vi "复制模板.vi"(8 "error in":errorcluster, 10 "服务器地址":path, 11 "工单号":string) -> (0 "error out":errorcluster, 1 "参数存储地址":path, 3 "source path out":path)   [LabVIEW 2016]
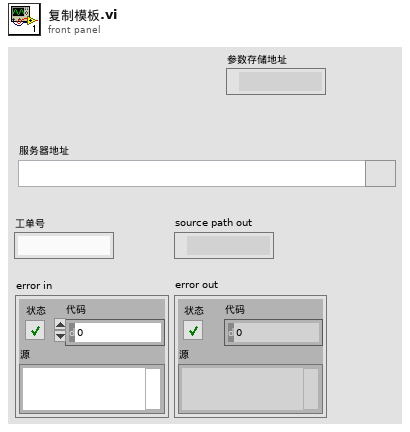
[diagram p1: front panel]
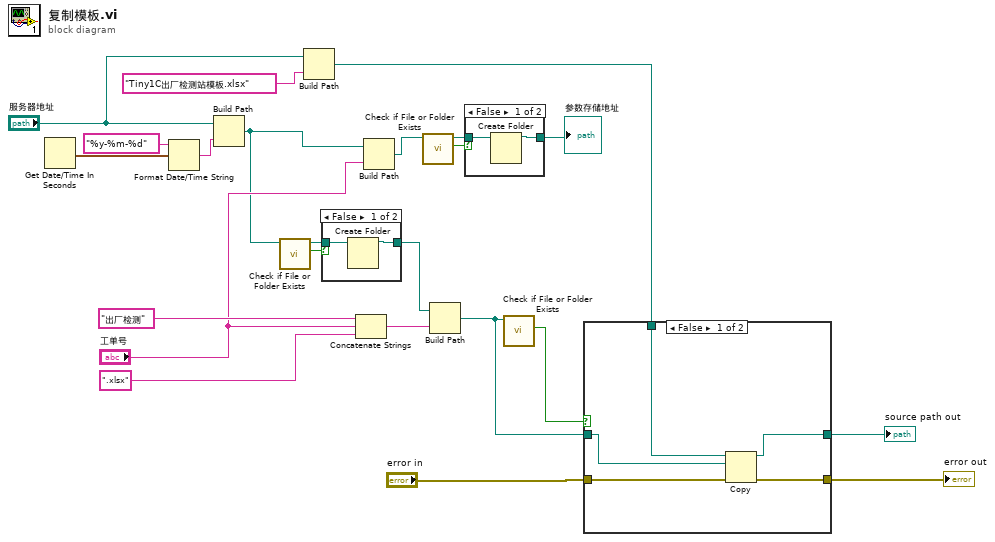
[diagram p0: block diagram]
diagram:
  n1 = Get Date/Time In Seconds() -> (seconds since 1Jan1904=w13:timestamp)
  n2 = Format Date/Time String(time format string (%c)="%y-%m-%d", seconds (now)=w13) -> (date/time string=w11:string)  [unwired: 1 in]
  n3 = Build Path(base path="服务器地址", name or relative path=w11) -> (appended path=w6:path)
  n4 = call <vilib>:"Check if File or Folder Exists.vi"("path"=w6) -> ("file or folder exists?"=w8:bool, "dup path"=w9:path)  [unwired: 8 in, 1 out]
  n5 = Build Path(base path="服务器地址", name or relative path="Tiny1C出厂检测站模板.xlsx") -> (appended path=w14:path)
  n6 = case shown="False" w8 {
    tunnel: w9 -> [w25 w26]
    tunnel: [w24 w26] -> w7
    frame False {
      n7 = Create Folder(path (use dialog)=w25) -> (created path=w24:path)  [unwired: 2 in, 2 out]
    }
    frame True {
    }
  }
  n8 = Concatenate Strings("出厂检测" ("string"), "工单号", ".xlsx" ("字符串")) -> (w23:string)
  n9 = Build Path(base path=w6, name or relative path="工单号") -> (appended path=w3:path)
  n10 = call <vilib>:"Check if File or Folder Exists.vi"("path"=w3) -> ("file or folder exists?"=w5:bool, "dup path"=w4:path)  [unwired: 8 in, 1 out]
  n11 = Build Path(base path=w7, name or relative path=w23) -> (appended path=w17:path)
  n12 = case shown="False" w5 {
    tunnel: w4 -> [w28 w29]
    tunnel: [w27 w29] -> w2
    frame False {
      n13 = Create Folder(path (use dialog)=w28) -> (created path=w27:path)  [unwired: 2 in, 2 out]
    }
    frame True {
    }
  }
  "参数存储地址" <- w2
  n14 = call <vilib>:"Check if File or Folder Exists.vi"("path"=w17) -> ("file or folder exists?"=w18:bool)  [unwired: 8 in, 2 out]
  n15 = case shown="False" w18 {
    tunnel: w14 -> [w34 _]
    tunnel: "error in" -> [w33 w36]
    tunnel: [w32 w36] -> w20
    tunnel: [w31 w35] -> w19
    tunnel: w17 -> [w30 w35]
    frame False {
      n16 = Copy(8:w33, 10:w30, 11:w34) -> (0:w32:errorcluster, 3:w31:path)  [unwired: 2 in, 1 out]
    }
    frame True {
    }
  }
  "error out" <- w20
  "source path out" <- w19
